vi "Controller LNLS Control PS Communication Loop.vi"(7 "Sync Objects":T1, 8 "error in (no error)":errorcluster, 11 "FOFB Configuration":T4={"FOFB Parameters"={"Network"={"FOFB Controller IP"="10.0.18.132", "LNLS Control Network IP"="10.0.18.132", "LNLS Control Network Power Supplies TCP Port"=4001, "LNLS Control Network FOFB Configuration TCP Port"=4002, "LNLS Control Network BPMs TCP Port"=4003, "Data Server TCP Port"=3600, "Monitoring Data TCP Port"=3601, "Configuration GUI TCP Port"=3602, "Storage Data TCP Port"=3603, "Fast Command TCP Port"=3604, "TCP Listening Timeout"=-1, "Request Setpoints Rate"=1000}, "Fast Acquisition"={"Acquisition Period"=320, "Data Buffer Size"=100, "Monitoring Period"=400000}, "Response Matrix Measurement"={"Step Amplitude"=0.65, "Time Between Steps"=1000, "Step Duration"=2000, "Number of Averages"=100}, "Correction Algorithm"={"Correction Period"=320, "Reference Orbit Path"=path "c:/fofb/Orbit/Referencia.orb", "Response Matrix Path"=path "c:/fofb/Response Matrix/Identity Matrix.resp", "Correction Matrix Path"=path "c:/fofb/Correction Matrix/Identity Matrix.corr", "PID Horizontal Gain"=0.005, "PID Vertical Gain"=0.005, "PID Horizontal Integral Time"=0.00066, "PID Vertical Integral Time"=0.00066, "PID Horizontal Derivative Time"=0.00066, "PID Vertical Derivative Time"=0.00066, "Beam Current FOFB Threshold"=10.0, "Decouple H-V"=TRUE, "Use Additional BPM LPF"=FALSE, "BPM LPF Cutoff"=10.0}, "Acquisition Network"=[], "Actuation Network"=[{"Chassis Name"="PS-RA01B", "Variables"=[{"Variable Name"="ACH01B", "Matrix Order"=1, "RMM Step Factor"=1.0, "Plane"=enum."H", "On Correction"=TRUE, "Kc"=0.0, "Ti"=0.0, "Td"=0.0}, {"Variable Name"="ACV01B", "Matrix Order"=4, "RMM Step Factor"=1.0, "Plane"=enum."V", "On Correction"=TRUE, "Kc"=0.0, "Ti"=0.0, "Td"=0.0}, {"Variable Name"="ACH03A", "Matrix Order"=3, "RMM Step Factor"=1.0, "Plane"=enum."H", "On Correction"=TRUE, "Kc"=0.0, "Ti"=0.0, "Td"=0.0}, {"Variable Name"="ACV03A", "Matrix Order"=7, "RMM Step Factor"=1.0, "Plane"=enum."V", "On Correction"=TRUE, "Kc"=0.0, "Ti"=0.0, "Td"=0.0}, {"Variable Name"="ALV02A", "Matrix Order"=5, "RMM Step Factor"=2.5, "Plane"=enum."V", "On Correction"=TRUE, "Kc"=0.0, "Ti"=0.0, "Td"=0.0}, {"Variable Name"="ALV02B", "Matrix Order"=6, "RMM Step Factor"=2.5, "Plane"=enum."V", "On Correction"=TRUE, "Kc"=0.0, "Ti"=0.0, "Td"=0.0}, {"Variable Name"="ACH02", "Matrix Order"=2, "RMM Step Factor"=1.0, "Plane"=enum."H", "On Correction"=TRUE, "Kc"=0.0, "Ti"=0.0, "Td"=0.0}]}]}, "Number of Acquisition Chassis"=1, "Number of Actuation Chassis"=1, "Number of BPM Readings"=7, "BPM Reading Names"=["ACH01B", "ACH02", "ACH03A", "ACV01B", "ALV02A", "ALV02B", "ACV03A"], "Selected BPM Readings"=[], "Number of Correctors"=7, "Corrector Names"=["ACH01B", "ACH02", "ACH03A", "ACV01B", "ALV02A", "ALV02B", "ACV03A"], "Selected Correctors"=[0, 1, 2, 3, 4, 5, 6], "Reference Orbit"=[-1.09330819, 0.83238826, -1.93923182, -0.39618552, -0.98307235, -1.88049663, 1.00296681, -0.19883275, -1.65005616, -0.55712353, 0.68544531, -0.70274756, -0.65496658, 0.05515979, -0.38935, 0.30350319, -0.13918837, -0.00011801, -0.21517587, -0.53815631, 0.44595451, 0.75898104, -0.44725813, -1.09971674, -0.46972415, -0.36841134, -0.07750092, 0.48295386, 0.47744403, 2.130847, 0.4681161, 0.39999255, -0.15570575, 0.89687682, 0.94383742, 1.1290593, -0.75786475, 0.54152616, 0.43217361, 0.98547068, 0.07993329, 0.29159442, 0.45045343, 0.73064824, 0.57741329, 0.86763439, 1.47745915, 1.05383194, 0.75658237, 0.2512502], "Response Matrix"=[[1.0, 1.0, 1.0, 1.0, 1.0, 1.0, 1.0], [1.0, 1.0, 1.0, 1.0, 1.0, 1.0, 1.0], [1.0, 1.0, 1.0, 1.0, 1.0, 1.0, 1.0], [1.0, 1.0, 1.0, 1.0, 1.0, 1.0, 1.0], [1.0, 1.0, 1.0, 1.0, 1.0, 1.0, 1.0], [1.0, 1.0, 1.0, 1.0, 1.0, 1.0, 1.0], [1.0, 1.0, 1.0, 1.0, 1.0, 1.0, 1.0]], "Correction Matrix"=[], "Acquisition Chassis Names"=["PS-RA01B (Cloned)"], "Actuation Chassis Names"=["PS-RA01B"], "Acquisition Variables"=[{"Variable Name"="ACH01B", "Chassis Name"="PS-RA01B (Cloned)"}, {"Variable Name"="ACH02", "Chassis Name"="PS-RA01B (Cloned)"}, {"Variable Name"="ACH03A", "Chassis Name"="PS-RA01B (Cloned)"}, {"Variable Name"="ACV01B", "Chassis Name"="PS-RA01B (Cloned)"}, {"Variable Name"="ALV02A", "Chassis Name"="PS-RA01B (Cloned)"}, {"Variable Name"="ALV02B", "Chassis Name"="PS-RA01B (Cloned)"}, {"Variable Name"="ACV03A", "Chassis Name"="PS-RA01B (Cloned)"}], "Actuation Variables"=[{"Variable Name"="ACH01B", "Chassis Name"="PS-RA01B"}, {"Variable Name"="ACH02", "Chassis Name"="PS-RA01B"}, {"Variable Name"="ACH03A", "Chassis Name"="PS-RA01B"}, {"Variable Name"="ACV01B", "Chassis Name"="PS-RA01B"}, {"Variable Name"="ALV02A", "Chassis Name"="PS-RA01B"}, {"Variable Name"="ALV02B", "Chassis Name"="PS-RA01B"}, {"Variable Name"="ACV03A", "Chassis Name"="PS-RA01B"}], "PS Matrix Mapping"=[{[0, 3, 2, 6, 4, 5, 1]}], "Inverse PS Matrix Mapping"=[[0, 0], [0, 6], [0, 2], [0, 1], [0, 4], [0, 5], [0, 3]], "BPM Matrix Mapping"=[{[0, 3, 2, 6, 4, 5, 1]}], "Inverse BPM Matrix Mapping"=[[0, 0], [0, 6], [0, 2], [0, 1], [0, 4], [0, 5], [0, 3]], "Response Matrix Beam Energy (MeV)"=0.0, "PID Parameters"=[{"Kc"=0.0, "Ti"=0.0, "Td"=0.0}, {"Kc"=0.0, "Ti"=0.0, "Td"=0.0}, {"Kc"=0.0, "Ti"=0.0, "Td"=0.0}, {"Kc"=0.0, "Ti"=0.0, "Td"=0.0}, {"Kc"=0.0, "Ti"=0.0, "Td"=0.0}, {"Kc"=0.0, "Ti"=0.0, "Td"=0.0}, {"Kc"=0.0, "Ti"=0.0, "Td"=0.0}], "BPM Planes"=[], "Corrector Planes"=[enum."H", enum."H", enum."H", enum."V", enum."V", enum."V", enum."V"], "RMM Step Factor"=[1.0, 1.0, 1.0, 1.0, 2.5, 2.5, 1.0]}) -> (0 "error out":errorcluster)   [LabVIEW 2011, in "Controller VIs.lvlib"]
uses:
  Controller VIs.lvlib
  Types Definitions/Type FOFB Configuration.ctl
  Types Definitions/Type FOFB Parameters.ctl
  Types Definitions/Type Network Configuration.ctl
  Types Definitions/Type FA Configuration.ctl
  Types Definitions/Type Response Matrix Measurement Configuration.ctl
  Types Definitions/Type Correction Algorithm Configuration.ctl
  Types Definitions/Type Acquisition Network Configuration.ctl
  Types Definitions/Type Actuation Network Configuration.ctl
  Types Definitions/Type PID Parameters.ctl
  Types Definitions/Type Synchronization Objects.ctl
  Types Definitions/Type Blocking Synchronization Objects.ctl
  Types Definitions/Type Monitoring Data.ctl
  Types Definitions/Type Operation Mode State.ctl
  Types Definitions/Type Diagnostics Data.ctl
  Types Definitions/Type CPU Loads Array.ctl
  Types Definitions/Type CPU Loads.ctl
  Types Definitions/Type Non-blocking Synchronization Objects.ctl
  Types Definitions/Type FOFB Variables.ctl
  Types Definitions/Type Actuation State.ctl
  Types Definitions/Type TCP State.ctl
  <vilib>/Platform/TimedLoop/XDataNode/timing_clust.ctl
  <vilib>/Platform/TimedLoop/XDataNode/nitl_modes.ctl
  <vilib>/Platform/TimedLoop/XDataNode/wakeup.ctl
  Controller Global Variables/Monitoring Data.vi
  <vilib>/Platform/TimedLoop/XDataNode/XDataNode.xnode
  LNLS Control VIs.lvlib
  Common VIs.lvlib
  Misc VIs.lvlib
  Controller Global Variables.lvlib
  <vilib>/Platform/TimedLoop/XDataNode/XDNodeRunTimeDep.lvlib
  Type Definitions.lvlib
panel:
  in  "send":bool
  in  "PS Status (On correction?)":bool[](array[boolean])=[FALSE, FALSE, FALSE, FALSE, FALSE, FALSE, FALSE]
  in  "PS Status (ON/OFF)":bool[](array[boolean])=[FALSE, FALSE, FALSE, FALSE, FALSE, FALSE, FALSE]
  in  "PS Setpoints":dbl[](array[numeric])=[0.0, 0.0, 0.0, 0.0, 0.0, 0.0, 0.0]
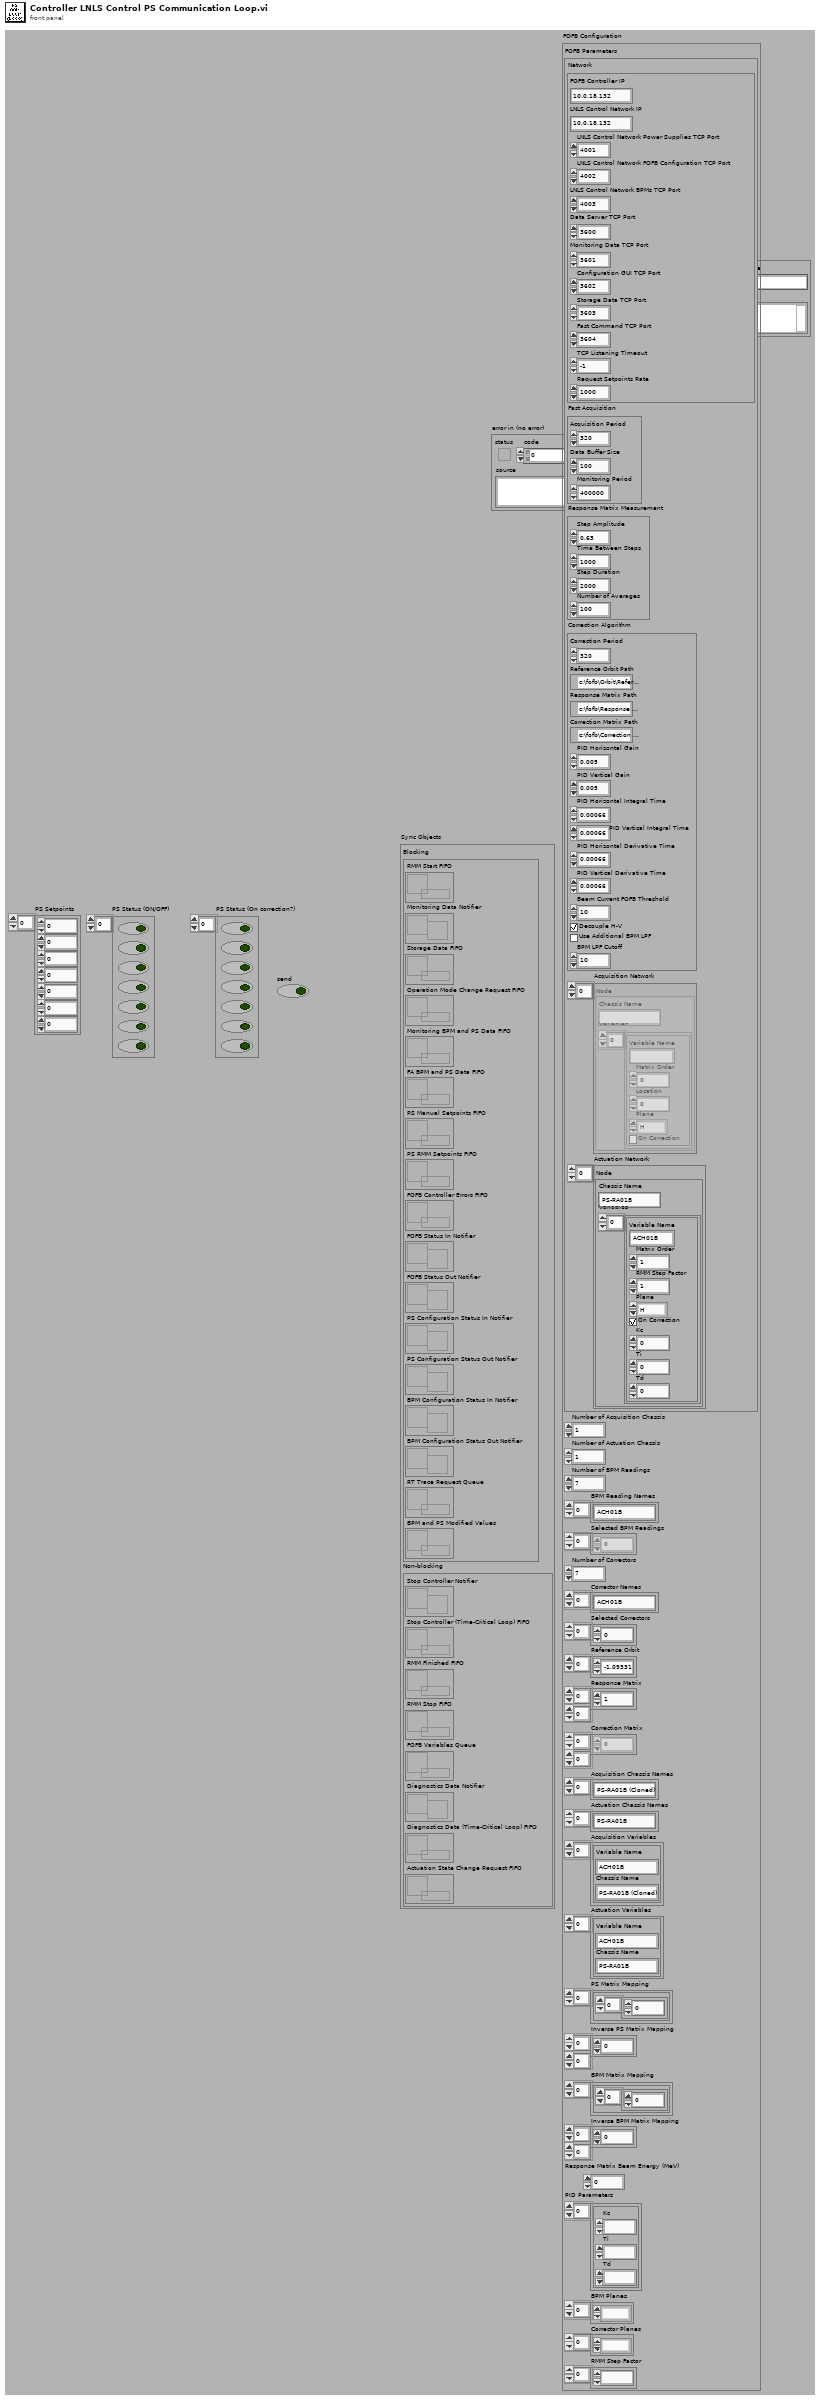
[diagram p1: front panel]
types:
  T1 = typedef "Type Definitions.lvlib/Type Synchronization Objects.ctl" = cluster{"Blocking":T2, "Non-blocking":T3}
  T2 = typedef "Type Definitions.lvlib/Type Blocking Synchronization Objects.ctl" = cluster{"RMM Start FIFO":refnum<k33>, "Monitoring Data Notifier":refnum<notifier>, "Storage Data FIFO":refnum<queue>, "Operation Mode Change Request FIFO":refnum<k33>, "Monitoring BPM and PS Data FIFO":refnum<k33>, "FA BPM and PS Data FIFO":refnum<k33>, "PS Manual Setpoints FIFO":refnum<k33>, "PS RMM Setpoints FIFO":refnum<k33>, "FOFB Controller Errors FIFO ":refnum<k33>, "FOFB Status In Notifier":refnum<notifier>, "FOFB Status Out Notifier":refnum<notifier>, "PS Configuration Status In Notifier":refnum<notifier>, "PS Configuration Status Out Notifier":refnum<notifier>, "BPM Configuration Status In Notifier":refnum<notifier>, "BPM Configuration Status Out Notifier":refnum<notifier>, "RT Trace Request Queue":refnum<queue>, "BPM and PS Modified Values":refnum<k33>}
  T3 = typedef "Type Definitions.lvlib/Type Non-blocking Synchronization Objects.ctl" = cluster{"Stop Controller Notifier":refnum<notifier>, "Stop Controller (Time-Critical Loop) FIFO":refnum<k33>, "RMM Finished FIFO":refnum<k33>, "RMM Stop FIFO":refnum<k33>, "FOFB Variables Queue":refnum<queue>, "Diagnostics Data Notifier":refnum<notifier>, "Diagnostics Data (Time-Critical Loop) FIFO":refnum<k33>, "Actuation State Change Request FIFO":refnum<k33>}
  T4 = typedef "Type Definitions.lvlib/Type FOFB Configuration.ctl" = cluster{"FOFB Parameters":T5, "Number of Acquisition Chassis":i32, "Number of Actuation Chassis":i32, "Number of BPM Readings":i32, "BPM Reading Names":string[], "Selected BPM Readings":u32[], "Number of Correctors":i32, "Corrector Names":string[], "Selected Correctors":u32[], "Reference Orbit":dbl[], "Response Matrix":dbl[][], "Correction Matrix":dbl[][], "Acquisition Chassis Names":string[], "Actuation Chassis Names":string[], "Acquisition Variables":cluster{"Variable Name":string, "Chassis Name":string}[], "Actuation Variables":cluster{"Variable Name":string, "Chassis Name":string}[], "PS Matrix Mapping":cluster{u32[]}[], "Inverse PS Matrix Mapping":u32[][], "BPM Matrix Mapping":cluster{u32[]}[], "Inverse BPM Matrix Mapping":u32[][], "Response Matrix Beam Energy (MeV)":dbl, "PID Parameters":T12[], "BPM Planes":enum8{"H", "V"}[], "Corrector Planes":enum8{"H", "V"}[], "RMM Step Factor":dbl[]}
  T5 = typedef "Type Definitions.lvlib/Type FOFB Parameters.ctl" = cluster{"Network":T6, "Fast Acquisition":T7, "Response Matrix Measurement":T8, "Correction Algorithm":T9, "Acquisition Network":T10, "Actuation Network":T11}
  T6 = typedef "Type Definitions.lvlib/Type Network Configuration.ctl" = cluster{"FOFB Controller IP":string, "LNLS Control Network IP":string, "LNLS Control Network Power Supplies TCP Port":u16, "LNLS Control Network FOFB Configuration TCP Port":u16, "LNLS Control Network BPMs TCP Port":u16, "Data Server TCP Port":u16, "Monitoring Data TCP Port":u16, "Configuration GUI TCP Port":u16, "Storage Data TCP Port":u16, "Fast Command TCP Port":u16, "TCP Listening Timeout":i32, "Request Setpoints Rate":u16}
  T7 = typedef "Type Definitions.lvlib/Type FA Configuration.ctl" = cluster{"Acquisition Period":u32, "Data Buffer Size":u32, "Monitoring Period":u32}
  T8 = typedef "Type Definitions.lvlib/Type Response Matrix Measurement Configuration.ctl" = cluster{"Step Amplitude":dbl, "Time Between Steps":u32, "Step Duration":u32, "Number of Averages":u32}
  T9 = typedef "Type Definitions.lvlib/Type Correction Algorithm Configuration.ctl" = cluster{"Correction Period":u32, "Reference Orbit Path":path, "Response Matrix Path":path, "Correction Matrix Path":path, "PID Horizontal Gain":dbl, "PID Vertical Gain":dbl, "PID Horizontal Integral Time":dbl, "PID Vertical Integral Time":dbl, "PID Horizontal Derivative Time":dbl, "PID Vertical Derivative Time":dbl, "Beam Current FOFB Threshold":dbl, "Decouple H-V":bool, "Use Additional BPM LPF":bool, "BPM LPF Cutoff":dbl}
  T10 = typedef "Type Definitions.lvlib/Type Acquisition Network Configuration.ctl" = cluster{"Chassis Name":string, "Variables":cluster{"Variable Name":string, "Matrix Order":u32, "Location":dbl, "Plane":enum8{"H", "V"}, "On Correction":bool}[]}[]
  T11 = typedef "Type Definitions.lvlib/Type Actuation Network Configuration.ctl" = cluster{"Chassis Name":string, "Variables":cluster{"Variable Name":string, "Matrix Order":u32, "RMM Step Factor":dbl, "Plane":enum8{"H", "V"}, "On Correction":bool, "Kc":dbl, "Ti":dbl, "Td":dbl}[]}[]
  T12 = typedef "Type Definitions.lvlib/Type PID Parameters.ctl" = cluster{"Kc":fxp<+/-,16,8>, "Ti":fxp<+/-,16,8>, "Td":fxp<+/-,16,8>}
  T13 = typedef "Type Definitions.lvlib/Type TCP State.ctl" = enum16{"Idle", "Wait Connection", "Read Data", "Process Data", "Write Data", "Close Connection"}
  T14 = typedef "XDNodeRunTimeDep.lvlib/timing_clust.ctl" = cluster{"Expected End [f-1]":u64, "Actual End [f-1]":u64, "Finished Late? [f-1]":bool, "Expected End [i-1]":u64, "Actual End [i-1]":u64, "Finished Late? [i-1]":bool, "Expected Start [i]":u64, "Actual Start [i]":u64, "Expected Start [f]":u64, "Actual Start [f]":u64, "Source Name":string, "Structure Name":string, "Period":i64, "Deadline":i64, "Offset":i64, "Start":i64, "Priority":i32, "Timeout":i32, "Mode":T15, "Wakeup Reason":T16, "Error":errorcluster, "Source Type":string, "Secondary Source Type":string, "Global End Time":u64, "Global Start Time":u64, "Frame Duration":u64, "Iteration Duration":u64, "Assigned CPU":i32, "I/O Scan Engine Mode":u32}
  T15 = typedef "XDNodeRunTimeDep.lvlib/nitl_modes.ctl" = enum32{"No Change", "Process missed periods, maintain original phase", "Discard missed periods, maintain original phase", "Process missed periods, ignore original phase", "Discard missed periods, ignore original phase"}
  T16 = typedef "XDNodeRunTimeDep.lvlib/wakeup.ctl" = enum32{"Normal", "Aborted", "Asynchronous wakeup", "Timing source error", "Timed loop error", "Timeout"}
  T17 = typedef "Type Definitions.lvlib/Type Monitoring Data.ctl" = cluster{"Timestamp":timestamp, "BPM Readings":dbl[], "PS Readings":dbl[], "PS FOFB Setpoints":dbl[], "PS Status per Rack":u8[], "PS ON-OFF per Rack":u8[], "Operation Mode":T18, "Diagnostics Data":T19, "Controller Status Table":i32[]}
  T18 = typedef "Type Definitions.lvlib/Type Operation Mode State.ctl" = enum8{"Idle Mode", "Manual Mode", "FOFB Mode", "RMM Mode"}
  T19 = typedef "Type Definitions.lvlib/Type Diagnostics Data.ctl" = cluster{"Time-Critical Loop Missed Iterations":u32, "Time-Critical Loop Execution Time (usec)":u32, "Available Memory (bytes)":u32, "CPU Loads Array":T20}
  T20 = typedef "Type Definitions.lvlib/Type CPU Loads Array.ctl" = T21[]
  T21 = typedef "Type Definitions.lvlib/Type CPU Loads.ctl" = cluster{"Total (%)":dbl, "Time Critical (%)":dbl, "Timed Structures (%)":dbl, "High (%)":dbl, "Above Normal (%)":dbl, "Normal (%)":dbl, "Background (%)":dbl, "Idle (%)":dbl, "ISR (%)":dbl}
  T22 = typedef "Type Definitions.lvlib/Type LOCON_BIPOLAR_16BITS.ctl" = cluster{"priority":u8, "flags":u8, "analog value":u16, "status":u8}
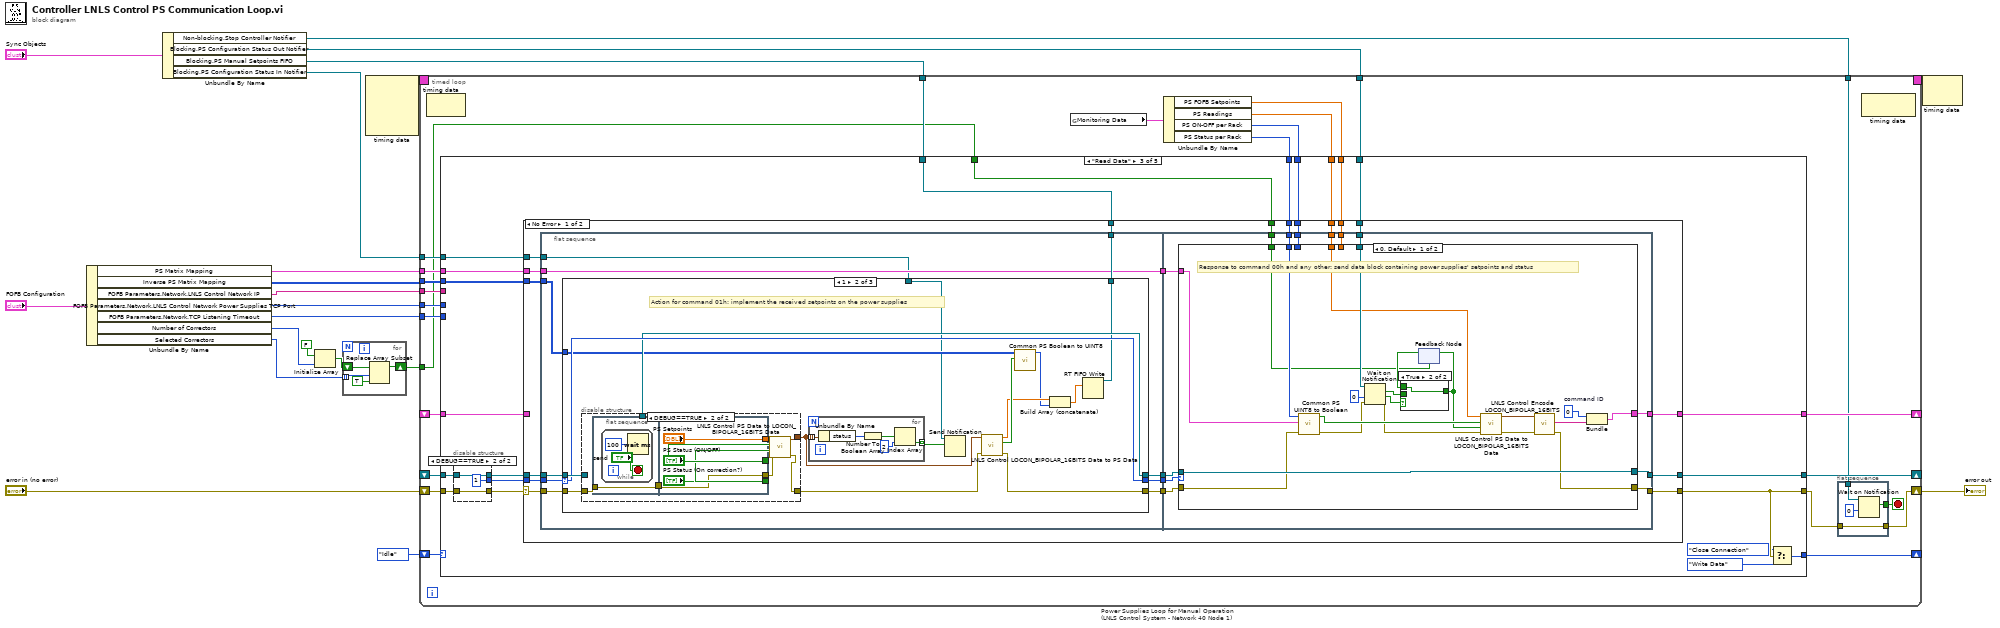
[diagram p0: block diagram]
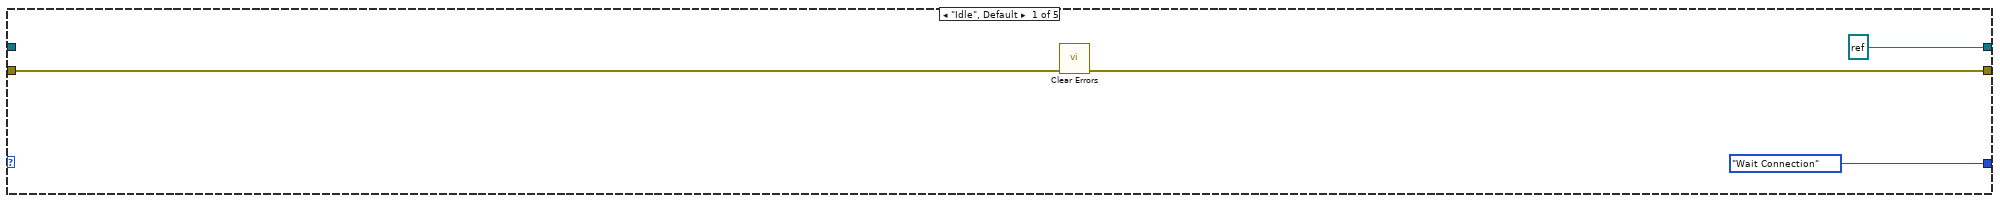
[diagram p2: hidden frame]
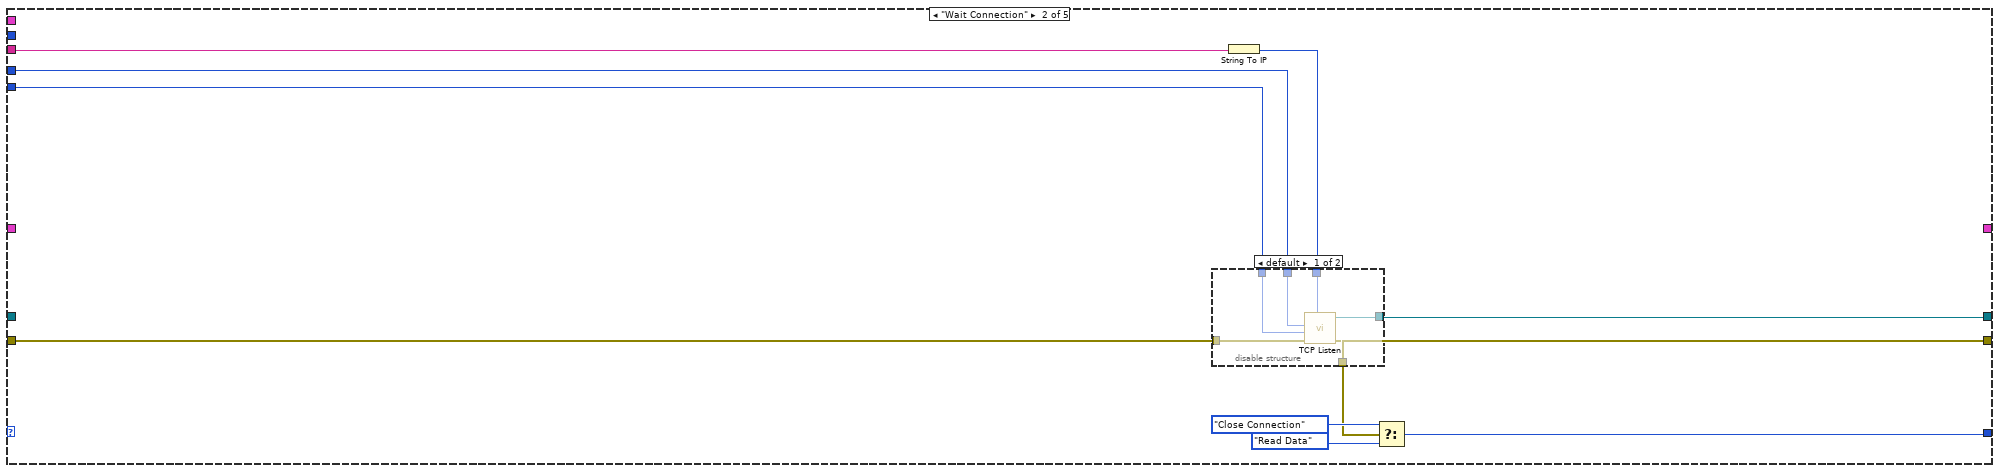
[diagram p3: hidden frame]
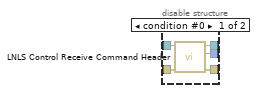
[diagram p5: hidden frame]
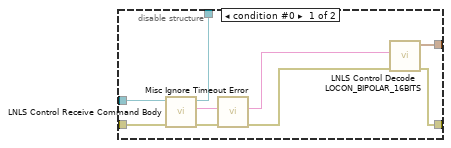
[diagram p7: hidden frame]
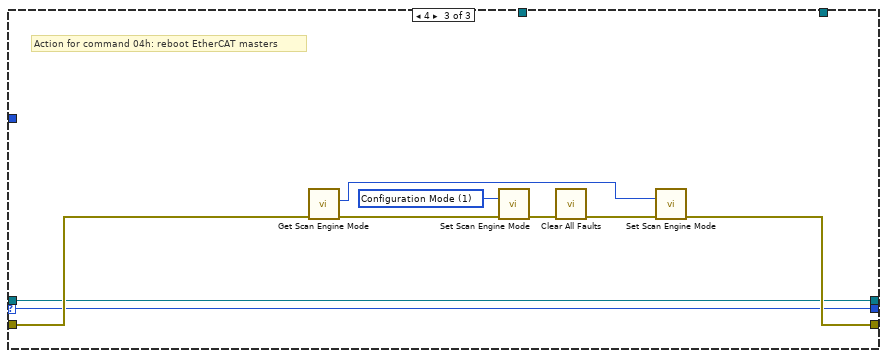
[diagram p8: hidden frame]
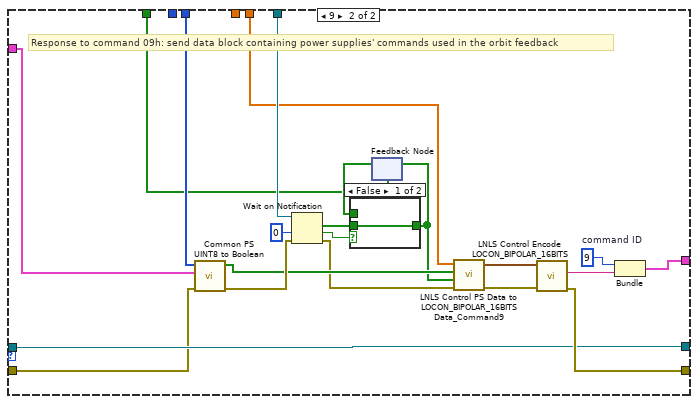
[diagram p10: hidden frame]
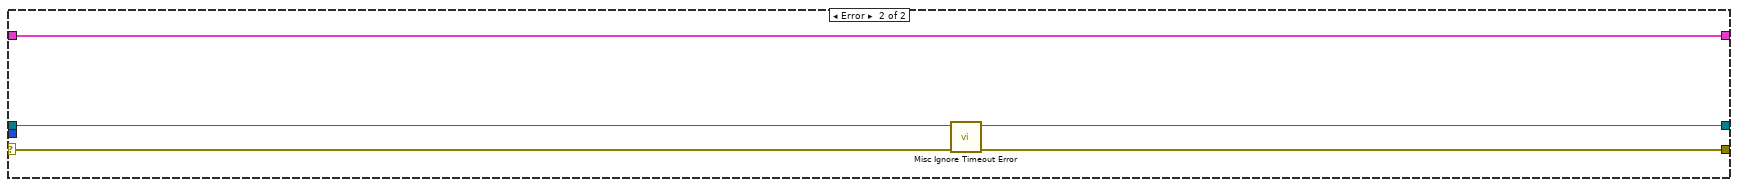
[diagram p12: hidden frame]
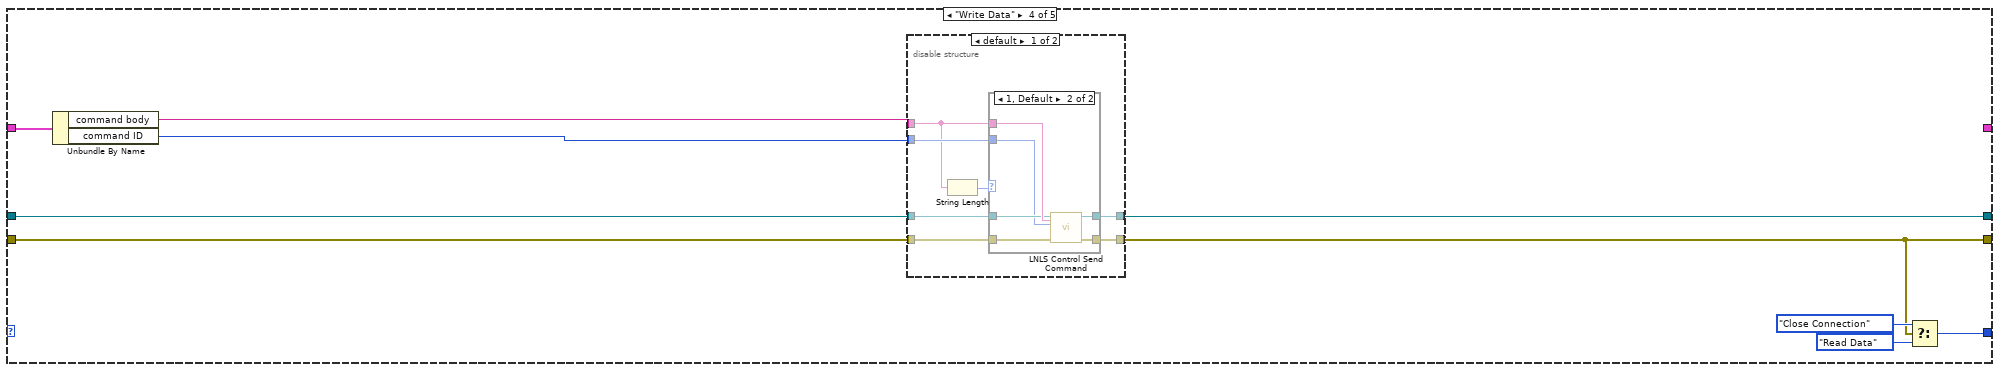
[diagram p13: hidden frame]
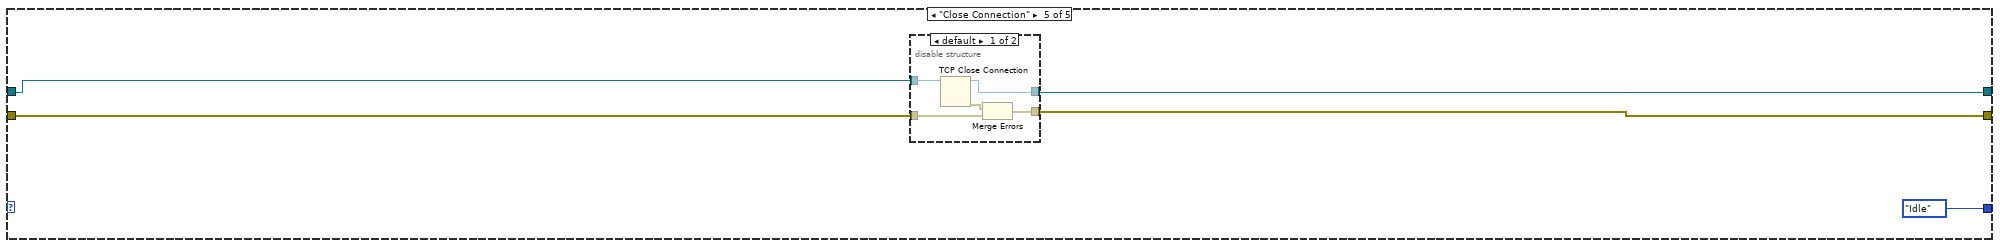
[diagram p16: hidden frame]
diagram:
  n1 = Unbundle By Name("FOFB Configuration") -> ("PS Matrix Mapping"=w14:cluster{u32[]}[], "Inverse PS Matrix Mapping"=w15:u32[][], "FOFB Parameters.Network.LNLS Control Network IP"=w16:string, "FOFB Parameters.Network.LNLS Control Network Power Supplies TCP Port"=w13:u16, "FOFB Parameters.Network.TCP Listening Timeout"=w11:i32, "Number of Correctors"=w5:i32, "Selected Correctors"=w3:u32[])
  n2 = Unbundle By Name("Sync Objects") -> ("Non-blocking.Stop Controller Notifier"=w12:refnum<notifier>, "Blocking.PS Configuration Status Out Notifier"=w8:refnum<notifier>, "Blocking.PS Manual Setpoints FIFO"=w1:refnum<k33>, "Blocking.PS Configuration Status In Notifier"=w7:refnum<notifier>)
  n3 = Initialize Array(FALSE, w5) -> (w4:bool[])
  n4 = for {
    tunnel: w3 -> [w25] mode=indexing
    shift-right: [w22] -> w2
    shift-left: w4 -> [w24]
    n5 = Replace Array Subset(array=w24, new element=TRUE ("new element/subarray"), index=w25) -> (w22:bool[])
  }
  n6 = node-c288() -> (w10:T14)  [unwired: 4 in]
  n7 = timed-loop "Power Supplies Loop for Manual Operation (LNLS Control System - Network 40 Node 1)" {
    shift-right: [w48] -> _
    shift-left: Type_TCP_State."Idle" ("f") -> [w50]
    shift-right: [w49] -> _
    shift-left: _ -> [w47]
    shift-right: [w35] -> w19
    shift-left: "error in (no error)" -> [w43]
    shift-right: [w45] -> _
    shift-left: _ -> [w44]
    tunnel: w13 -> [w46]
    tunnel: w16 -> [w42]
    tunnel: w15 -> [w41]
    tunnel: w14 -> [w40]
    tunnel: w12 -> [w38]
    tunnel: w11 -> [w39]
    tunnel: w1 -> [w31]
    timing: w10 -> [_]
    timing-out: [_] -> w9
    tunnel: w8 -> [w28]
    tunnel: w7 -> [w27]
    tunnel: w2 -> [w26]
    stop <- w37 stop-if-true
    n8 = node-c288() -> ()  [unwired: 1 in, 1 out]
    n9 = global read "Monitoring Data.vi" "Monitoring Data"() -> (w32:T17)
    n10 = Unbundle By Name(w32) -> ("PS FOFB Setpoints"=w34:dbl[], "PS Readings"=w33:dbl[], "PS ON-OFF per Rack"=w29:u8[], "PS Status per Rack"=w30:u8[])
    n11 = case shown="\"Read Data\"" w50 {
      tunnel: [refnum<k5> refnum ("connection ID") w67 w99 w259 w286] -> w49
      tunnel: [w58 w62 w97 w258 w283] -> w36
      tunnel: [Type_TCP_State."Wait Connection" w70 w98 w263 Type_TCP_State."Idle"] -> w48
      tunnel: w47 -> [_ _ w95 w261 w287]
      tunnel: w43 -> [w57 w63 w96 w260 w284]
      tunnel: w46 -> [_ w66 _ _ _]
      tunnel: [_ _ w92 _ _] -> w45
      tunnel: w44 -> [_ _ w90 w262 _]
      tunnel: w42 -> [_ w64 _ _ _]
      tunnel: w41 -> [_ _ w88 _ _]
      tunnel: w40 -> [_ _ w87 _ _]
      tunnel: w39 -> [_ w61 _ _ _]
      tunnel: w34 -> [_ _ w78 _ _]
      tunnel: w33 -> [_ _ w79 _ _]
      tunnel: w30 -> [_ _ w86 _ _]
      tunnel: w31 -> [_ _ w85 _ _]
      tunnel: w29 -> [_ _ w84 _ _]
      tunnel: w28 -> [_ _ w83 _ _]
      tunnel: w27 -> [_ _ w81 _ _]
      tunnel: w26 -> [_ _ w80 _ _]
      frame "Idle", Default {
        n12 = call <vilib>:"Clear Errors.vi"("error in (no error)"=w57) -> ("error out"=w58:errorcluster)  [unwired: 6 in]
      }
      frame "Wait Connection" {
        n13 = String To IP(1:w64) -> (0:w65:u32)
        n14 = disable-structure shown="default" {
          disable-tunnel: [w76 _] -> w67
          disable-tunnel: w66 -> [w75 _]
          disable-tunnel: w65 -> [w74 _]
          disable-tunnel: w63 -> [w73 w77]
          disable-tunnel: [w72 w77] -> w62
          disable-tunnel: w61 -> [w71 _]
          frame condition #0 {
            n15 = call <vilib>:"TCP Listen.vi"("net address"=w74, "error in (no error)"=w73, "timeout ms (wait forever: -1)"=w71, "port"=w75) -> ("error out"=w72:errorcluster, "connection ID"=w76:refnum<k5>)  [unwired: 3 in, 3 out]
          }
          frame condition #1 (active) {
          }
        }
        n16 = Select(t=Type_TCP_State."Close Connection", s=w62, f=Type_TCP_State."Read Data") -> (s? t:f=w70:T13)
      }
      frame "Read Data" {
        n17 = disable-structure shown="DEBUG==TRUE" {
          disable-tunnel: w96 -> [w104 w107]
          disable-tunnel: w95 -> [w103 w106]
          disable-tunnel: [w102 w106] -> w94
          disable-tunnel: [w101 w107] -> w91
          disable-tunnel: [w100 u8 1 ("command ID")] -> w82
          frame condition #0 {
            n18 = call "LNLS Control Receive Command Header.vi"("error in (no error)"=w104, "connection ID"=w103) -> ("error out"=w101:errorcluster, "command ID"=w100:u8, "connection ID out"=w102:refnum<k5>)  [unwired: 7 in]
          }
          frame condition #1 (active) {
          }
        }
        n19 = case shown="No Error" w91 {
          selector: w91 -> [w122 w252]
          tunnel: [w127 w255] -> w99
          tunnel: [w126 w253] -> w97
          tunnel: w94 -> [w125 w255]
          tunnel: w82 -> [w124 _]
          tunnel: [w123 w254] -> w92
          tunnel: w90 -> [_ w254]
          tunnel: w88 -> [w118 _]
          tunnel: w87 -> [w116 _]
          tunnel: w78 -> [w115 _]
          tunnel: w79 -> [w114 _]
          tunnel: w86 -> [w113 _]
          tunnel: w85 -> [w112 _]
          tunnel: w84 -> [w111 _]
          tunnel: w83 -> [w110 _]
          tunnel: w81 -> [w109 _]
          tunnel: w80 -> [w108 _]
          frame No Error {
            n20 = flat-sequence {
              tunnel: [w137] -> w121
              tunnel: [w136] -> w120
              tunnel: w125 -> [w135]
              tunnel: w124 -> [w134]
              tunnel: w122 -> [w133]
              tunnel: [w132] -> w119
              tunnel: w118 -> [w131]
              tunnel: [w129] -> w117
              tunnel: w116 -> [w129]
              tunnel: w112 -> [w130]
              tunnel: w109 -> [w128]
              tunnel: [w202] -> w127
              tunnel: w121 -> [w201]
              tunnel: [w205] -> w126
              tunnel: w120 -> [w204]
              tunnel: [w200] -> w123
              tunnel: w119 -> [w203]
              tunnel: w117 -> [w199]
              tunnel: w115 -> [w198]
              tunnel: w114 -> [w197]
              tunnel: w113 -> [w196]
              tunnel: w111 -> [w195]
              tunnel: w110 -> [w194]
              tunnel: w108 -> [w193]
              frame #0 {
                n21 = case shown="1" w134 {
                  selector: w134 -> [w138 w152 w185]
                  tunnel: w133 -> [w140 w154 w192]
                  tunnel: [w140 w153 w191] -> w136
                  tunnel: [w139 w151 w184] -> w137
                  tunnel: w135 -> [w139 w155 w184]
                  tunnel: [w138 w152 w185] -> w132
                  tunnel: w131 -> [_ w150 _]
                  tunnel: w130 -> [_ w148 _]
                  tunnel: w128 -> [_ w143 _]
                  frame 0, Default {
                  }
                  frame 1 {
                    # "Action for command 01h: implement the received setpoints on the power supplies"
                    n22 = disable-structure shown="DEBUG==TRUE" {
                      disable-tunnel: w155 -> [w163 _]
                      disable-tunnel: w154 -> [w162 w167]
                      disable-tunnel: [w161 _] -> w151
                      disable-tunnel: [w157 w171] -> w144
                      disable-tunnel: [w156 w165] -> w142
                      frame condition #0 {
                        n23 = call "LNLS Control Receive Command Body.vi"("error in (no error)"=w162, "connection ID"=w163) -> ("error out"=w158:errorcluster, "command body"=w159:string, "connection ID out"=w161:refnum<k5>)  [unwired: 6 in, 1 out]
                        n24 = call "Misc Ignore Timeout Error.vi"("error in (no error)"=w158) -> ("error out"=w160:errorcluster)  [unwired: 9 in, 1 out]
                        n25 = call "LNLS Control Decode LOCON_BIPOLAR_16BITS.vi"("error in (no error)"=w160, "command body"=w159) -> ("error out"=w156:errorcluster, "LOCON data"=w157:T22[])  [unwired: 6 in]
                      }
                      frame condition #1 (active) {
                        n26 = flat-sequence {
                          tunnel: w167 -> [w172]
                          tunnel: [w172] -> w164
                          tunnel: ["PS Setpoints"] -> w170
                          tunnel: ["PS Status (ON/OFF)"] -> w169
                          tunnel: ["PS Status (On correction?)"] -> w168
                          tunnel: [w175] -> w166
                          tunnel: w164 -> [w175]
                          frame #0 {
                            n27 = while {
                              stop <- "send" stop-if-true
                              n28 = Wait (ms)(milliseconds to wait=u32 100) -> ()  [unwired: 1 out]
                            }
                          }
                          frame #1 {
                          }
                        }
                        n29 = call "LNLS Control PS Data to LOCON_BIPOLAR_16BITS Data.vi"("error in (no error)"=w166, "PS Status (On correction?)"=w168, "PS Status (ON/OFF)"=w169, "PS Readings/Setpoints"=w170) -> ("error out"=w165:errorcluster, "PS Readings/Setpoints LOCON Data"=w171:T22[])  [unwired: 6 in]
                      }
                    }
                    n30 = for {
                      tunnel: w144 -> [w183] mode=indexing
                      tunnel: [w181] -> w141 mode=indexing
                      n31 = Unbundle By Name(w183) -> ("status"=w180:u8)
                      n32 = Number To Boolean Array(number=w180) -> (Boolean array=w179:bool[])
                      n33 = Index Array(array=w179, index=2) -> (element=w181:bool)
                    }
                    n34 = Send Notification(notification=w141, notifier=w143) -> ()  [unwired: 1 in, 2 out]
                    n35 = call "LNLS Control LOCON_BIPOLAR_16BITS Data to PS Data.vi"("error in (no error)"=w142, "PS Setpoints LOCON Data"=w144) -> ("error out"=w153:errorcluster, "PS Status"=w149:bool[], "PS Setpoints"=w147:dbl[])  [unwired: 7 in]
                    n36 = call "Common PS Boolean to UINT8.vi"("PS ON-OFF"=w149, "Inverse PS Matrix Mapping"=w150) -> ("PS ON-OFF (per PS Rack)"=w146:u8[])  [unwired: 8 in, 1 out]
                    n37 = Build Array (concatenate)(w147, w146) -> (w145:dbl[])
                    n38 = RT FIFO Write(0:w148, 1:w145) -> ()  [unwired: 3 in, 4 out]
                  }
                  frame 4 {
                    w190 = 1 items=["Configuration Mode"=1, "Active Mode"=2] ("mode (Active Mode)")
                    # "Action for command 04h: reboot EtherCAT masters"
                    n39 = call <vilib>:"Get Scan Engine Mode.vi"("error in (no error)"=w192) -> ("error out"=w189:errorcluster, "mode"=w186:i32)  [unwired: 9 in]
                    n40 = call <vilib>:"Set Scan Engine Mode.vi"("mode (Active Mode)"=w190, "error in (no error)"=w189) -> ("error out"=w188:errorcluster)  [unwired: 13 in]
                    n41 = call <vilib>:"Clear All Faults.vi"("error in (no error)"=w188) -> ("error out"=w187:errorcluster)  [unwired: 1 in, 9 out]
                    n42 = call <vilib>:"Set Scan Engine Mode.vi"("mode (Active Mode)"=w186, "error in (no error)"=w187) -> ("error out"=w191:errorcluster)  [unwired: 13 in]
                  }
                }
              }
              frame #1 {
                n43 = case shown="0, Default" w203 {
                  tunnel: w204 -> [w221 w244]
                  tunnel: [w222 w247] -> w205
                  tunnel: [w226 w246] -> w202
                  tunnel: w201 -> [w226 w246]
                  tunnel: [w223 w245] -> w200
                  tunnel: w199 -> [w220 w243]
                  tunnel: w198 -> [_ w234]
                  tunnel: w197 -> [w206 _]
                  tunnel: w196 -> [w218 _]
                  tunnel: w195 -> [_ w242]
                  tunnel: w194 -> [w215 w241]
                  tunnel: w193 -> [w207 w235]
                  frame 0, Default {
                    w224 = u8 0  # command ID
                    # "Response to command 00h and any other: send data block containing power supplies' setpoints and status"
                    n44 = call "Common PS UINT8 to Boolean.vi"("error in (no error)"=w221, "PS Matrix Mapping"=w220, "PS Status (per PS Rack)"=w218) -> ("error out"=w214:errorcluster, "PS Status"=w216:bool[])  [unwired: 7 in]
                    n45 = Wait on Notification(notifier=w215, timeout in ms (-1)=0, error in (no error)=w214) -> (notification=w211:bool[], timed out?=w212:bool, error out=w213:errorcluster)  [unwired: 1 in, 1 out]
                    n46 = feedback #1(w207) -> (w208:bool[])
                    n47 = case shown="True" w212 {
                      tunnel: w211 -> [w227 _]
                      tunnel: [w227 w228] -> w209
                      tunnel: w208 -> [_ w228]
                      frame False {
                      }
                      frame True {
                      }
                    }
                    n48 = feedback-in #1(w209) -> ()
                    n49 = call "LNLS Control PS Data to LOCON_BIPOLAR_16BITS Data.vi"("error in (no error)"=w213, "PS Status (On correction?)"=w209, "PS Status (ON/OFF)"=w216, "PS Readings/Setpoints"=w206) -> ("error out"=w225:errorcluster, "PS Readings/Setpoints LOCON Data"=w217:T22[])  [unwired: 6 in]
                    n50 = call "LNLS Control Encode LOCON_BIPOLAR_16BITS.vi"("error in (no error)"=w225, "LOCON Data"=w217) -> ("error out"=w222:errorcluster, "command body"=w219:string)  [unwired: 8 in]
                    n51 = Bundle("command ID"=w224, "command body"=w219) -> (w223:cluster{"command ID":u8, "command body":string})  [unwired: 1 in]
                  }
                  frame 9 {
                    w248 = u8 9  # command ID
                    # "Response to command 09h: send data block containing power supplies' commands used in the orbit feedback"
                    n52 = call "Common PS UINT8 to Boolean.vi"("error in (no error)"=w244, "PS Matrix Mapping"=w243, "PS Status (per PS Rack)"=w242) -> ("error out"=w240:errorcluster, "PS Status"=w233:bool[])  [unwired: 7 in]
                    n53 = Wait on Notification(notifier=w241, timeout in ms (-1)=0, error in (no error)=w240) -> (notification=w237:bool[], timed out?=w236:bool, error out=w231:errorcluster)  [unwired: 1 in, 1 out]
                    n54 = feedback #2(w235) -> (w238:bool[])
                    n55 = case shown="False" w236 {
                      tunnel: w237 -> [w250 _]
                      tunnel: [w250 w251] -> w232
                      tunnel: w238 -> [_ w251]
                      frame False {
                      }
                      frame True {
                      }
                    }
                    n56 = feedback-in #2(w232) -> ()
                    n57 = call "LNLS Control PS Data to LOCON_BIPOLAR_16BITS Data_Command9.vi"("error in (no error)"=w231, "PS Status (On correction?)"=w232, "PS Status (ON/OFF)"=w233, "PS Readings/Setpoints"=w234) -> ("error out"=w229:errorcluster, "PS Readings/Setpoints LOCON Data"=w230:T22[])  [unwired: 6 in]
                    n58 = call "LNLS Control Encode LOCON_BIPOLAR_16BITS.vi"("error in (no error)"=w229, "LOCON Data"=w230) -> ("error out"=w247:errorcluster, "command body"=w249:string)  [unwired: 8 in]
                    n59 = Bundle("command ID"=w248, "command body"=w249) -> (w245:cluster{"command ID":u8, "command body":string})  [unwired: 1 in]
                  }
                }
              }
            }
          }
          frame Error {
            n60 = call "Misc Ignore Timeout Error.vi"("error in (no error)"=w252) -> ("error out"=w253:errorcluster)  [unwired: 9 in, 1 out]
          }
        }
        n61 = Select(t=Type_TCP_State."Close Connection", s=w97, f=Type_TCP_State."Write Data") -> (s? t:f=w98:T13)
      }
      frame "Write Data" {
        n62 = Unbundle By Name(w262) -> ("command body"=w256:string, "command ID"=w257:u8)
        n63 = disable-structure shown="default" {
          disable-tunnel: w261 -> [w272 w281]
          disable-tunnel: w260 -> [w271 w282]
          disable-tunnel: [w270 w281] -> w259
          disable-tunnel: [w269 w282] -> w258
          disable-tunnel: w257 -> [w268 _]
          disable-tunnel: w256 -> [w266 _]
          frame condition #0 {
            n64 = String Length(string=w266) -> (length=w267:i32)
            n65 = case shown="1, Default" w267 {
              tunnel: w266 -> [_ w280]
              tunnel: w272 -> [w274 w279]
              tunnel: w271 -> [w273 w278]
              tunnel: [w274 w277] -> w270
              tunnel: [w273 w276] -> w269
              tunnel: w268 -> [_ w275]
              frame 0 {
              }
              frame 1, Default {
                n66 = call "LNLS Control Send Command.vi"("command body"=w280, "error in (no error)"=w278, "command ID"=w275, "connection ID"=w279) -> ("error out"=w276:errorcluster, "connection ID out"=w277:refnum<k5>)  [unwired: 6 in]
              }
            }
          }
          frame condition #1 (active) {
          }
        }
        n67 = Select(t=Type_TCP_State."Close Connection", s=w258, f=Type_TCP_State."Read Data") -> (s? t:f=w263:T13)
      }
      frame "Close Connection" {
        n68 = disable-structure shown="default" {
          disable-tunnel: w287 -> [w292 w293]
          disable-tunnel: [w291 w293] -> w286
          disable-tunnel: w284 -> [w290 w294]
          disable-tunnel: [w288 w294] -> w283
          frame condition #0 {
            n69 = TCP Close Connection(connection ID=w292) -> (connection ID out=w291:refnum<k5>, error out=w289:errorcluster)  [unwired: 2 in]
            n70 = Merge Errors(w289, w290) -> (w288:errorcluster)
          }
          frame condition #1 (active) {
          }
        }
      }
    }
    n71 = flat-sequence {
      tunnel: w38 -> [w55]
      tunnel: w36 -> [w53]
      tunnel: [w53] -> w35
      tunnel: [w54] -> w37
      frame #0 {
        n72 = Wait on Notification(notifier=w55, timeout in ms (-1)=0) -> (notification=w54:bool)  [unwired: 2 in, 3 out]
      }
    }
    n73 = node-c288() -> ()  [unwired: 1 in, 1 out]
  }
  "error out" <- w19
  n74 = node-c288(w9) -> ()  [unwired: 1 out]
